vi "aal_cascaded moving average.vi"   [LabVIEW 2012, in "NI_AALPro.lvlib"]
uses:
  NI_AALPro.lvlib
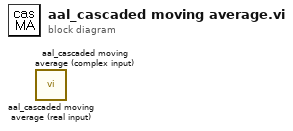
[diagram p0: block diagram]
diagram:
  n1 = call "aal_cascaded moving average (real input).vi"() -> ()  [unwired: 4 in, 1 out]
  n2 = call "aal_cascaded moving average (complex input).vi"() -> ()  [unwired: 4 in, 1 out]
